vi "Set Bundler Input Count.vi"(8 "error in (no error)":errorcluster, 10 "Numeric":i32, 11 "Bundler in":refnum<vi>) -> (0 "error out":errorcluster, 3 "Bundler out":refnum<vi>)   [LabVIEW 2019, in "gRPC Template Creation Utility.lvlib"]
uses:
  gRPC Template Creation Utility.lvlib
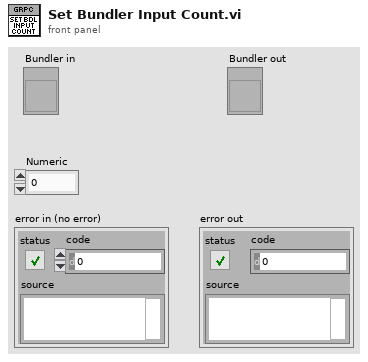
[diagram p1: front panel]
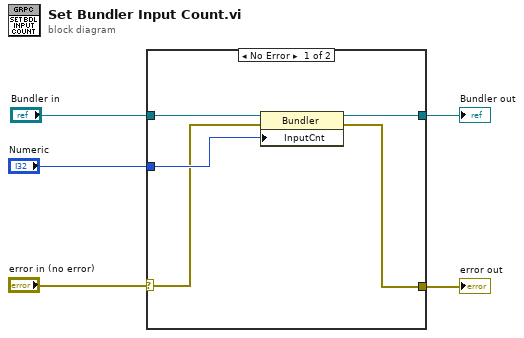
[diagram p0: block diagram]
diagram:
  n1 = case shown="No Error" "error in (no error)" {
    selector: "error in (no error)" -> [w6 w12]
    tunnel: [w10 w12] -> w5
    tunnel: [w9 w11] -> w1
    tunnel: "Bundler in" -> [w8 w11]
    tunnel: "Numeric" -> [w7 _]
    frame No Error {
      n2 = property class="Bundler"(reference=w8, error in=w6, "InputCnt"=w7) -> (reference out=w9:refnum<vi>, error out=w10:errorcluster)
    }
    frame Error {
    }
  }
  "error out" <- w5
  "Bundler out" <- w1
